vi "FTW-Ether-Destroy.vi"(5 "Force Destroy?":bool, 11 "error in":errorcluster) -> (15 "error out":errorcluster)   [LabVIEW 2015, in "FTW-Ether.lvclass"]
uses:
  FTW-Ether.lvclass
  EventLogger/FTW-Logger.lvclass
  FTW-Ether-Connections-Action.ctl
  Connector/FTW-ActorConnector.lvclass
  FTW-Ether-Instance.vi
panel:
  # "Inputs"
  # "Outputs"
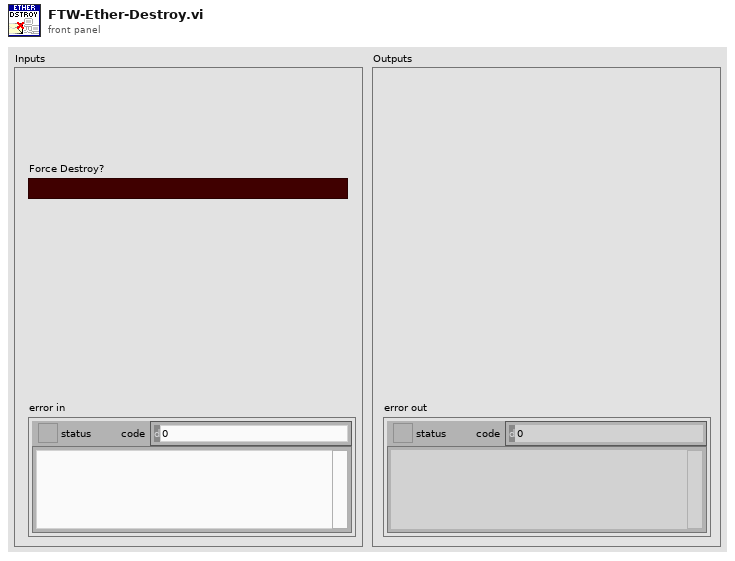
[diagram p1: front panel]
types:
  T1 = typedef "FTW-Ether.lvclass/FTW-Ether-Connections-Action.ctl" = enum8{"Query", "Add", "Reset"}
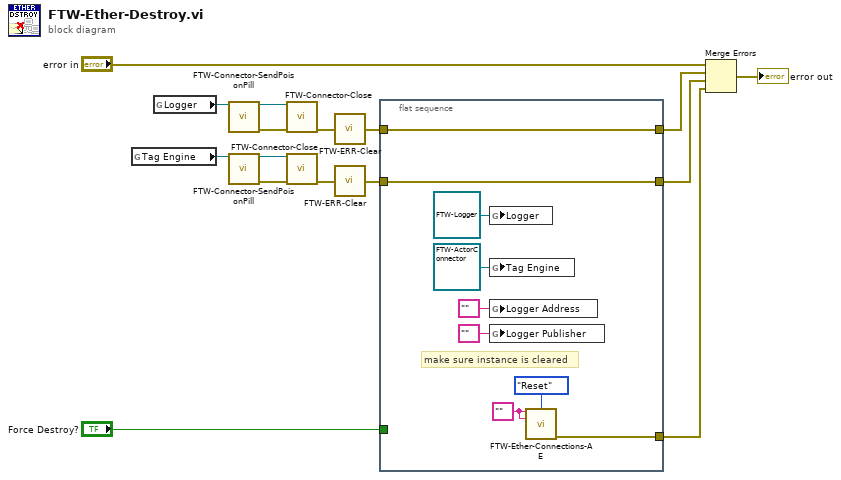
[diagram p0: block diagram]
diagram:
  n1 = global read "FTW-Ether-Instance.vi" "Tag Engine"() -> (w6:refnum<class "FTW-ActorConnector.lvclass">)
  n2 = global read "FTW-Ether-Instance.vi" "Logger"() -> (w8:refnum<class "FTW-Logger.lvclass">)
  n3 = call-dynamic "FTW-Connector-SendPoisonPill.vi"("FTW Actor Connector"=w8) -> ("FTW Actor Connector out"=w14:refnum<class "FTW-Logger.lvclass">, "error out"=w13:errorcluster)  [unwired: 9 in, 4 out]
  n4 = call-dynamic "FTW-Connector-SendPoisonPill.vi"("FTW Actor Connector"=w6) -> ("FTW Actor Connector out"=w3:refnum<class "FTW-ActorConnector.lvclass">, "error out"=w4:errorcluster)  [unwired: 9 in, 4 out]
  n5 = call-dynamic "FTW-Connector-Close.vi"("FTW Actor Connector"=w14, "error in"=w13) -> ("error out"=w10:errorcluster)  [unwired: 13 in]
  n6 = call-dynamic "FTW-Connector-Close.vi"("FTW Actor Connector"=w3, "error in"=w4) -> ("error out"=w5:errorcluster)  [unwired: 13 in]
  n7 = call "FTW-ERR-Clear.vi"("error to snuff"=w10) -> ("no error"=w9:errorcluster)
  n8 = call "FTW-ERR-Clear.vi"("error to snuff"=w5) -> ("no error"=w2:errorcluster)
  n9 = flat-sequence {
    tunnel: "Force Destroy?" -> [_]
    tunnel: w9 -> [w25]
    tunnel: [w25] -> w11
    tunnel: [w20] -> w7
    tunnel: [w18] -> w1
    tunnel: w2 -> [w18]
    frame #0 {
      w21 = "" ("empty string")
      # "make sure instance is cleared"
      n10 = global write "FTW-Ether-Instance.vi" "Logger"(refnum<class "FTW-Logger.lvclass"> refnum ("Logger")) -> ()
      n11 = global write "FTW-Ether-Instance.vi" "Tag Engine"(refnum<class "FTW-ActorConnector.lvclass"> refnum ("Tag Engine")) -> ()
      n12 = global write "FTW-Ether-Instance.vi" "Logger Address"("" ("Logger Address")) -> ()
      n13 = global write "FTW-Ether-Instance.vi" "Logger Publisher"("" ("Logger Address")) -> ()
      n14 = call "FTW-Ether-Connections-AE.vi"("Connection"=w21, "Action"=FTW-Ether-Connections-Action."Reset", "Address"=w21) -> ("error out"=w20:errorcluster)  [unwired: 11 in, 1 out]
    }
  }
  n15 = Merge Errors("error in", w11, w1, w7) -> (→"error out":errorcluster)
